vi "Eval Ping Feedback.vi"(7 "IP Address(loopback=127.0.0.1)":string="127.0.0.1", 8 "error in (no error)":errorcluster, 9 "Pings sent":i32, 10 "Ping feedback":string, 11 "object in":refnum<class "Ghetto_ping.lvclass">) -> (0 "error out":errorcluster, 1 "Report":string, 2 "Fraction returned":dbl, 3 "object out":refnum<class "Ghetto_ping.lvclass">)   [LabVIEW 2013, in "Ghetto_ping.lvclass"]
uses:
  Ghetto_ping.lvclass
panel:
  # "I AM REENTRANT"
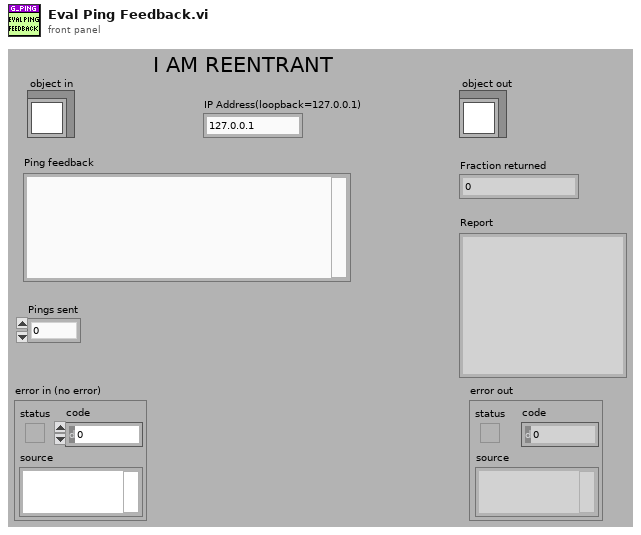
[diagram p1: front panel]
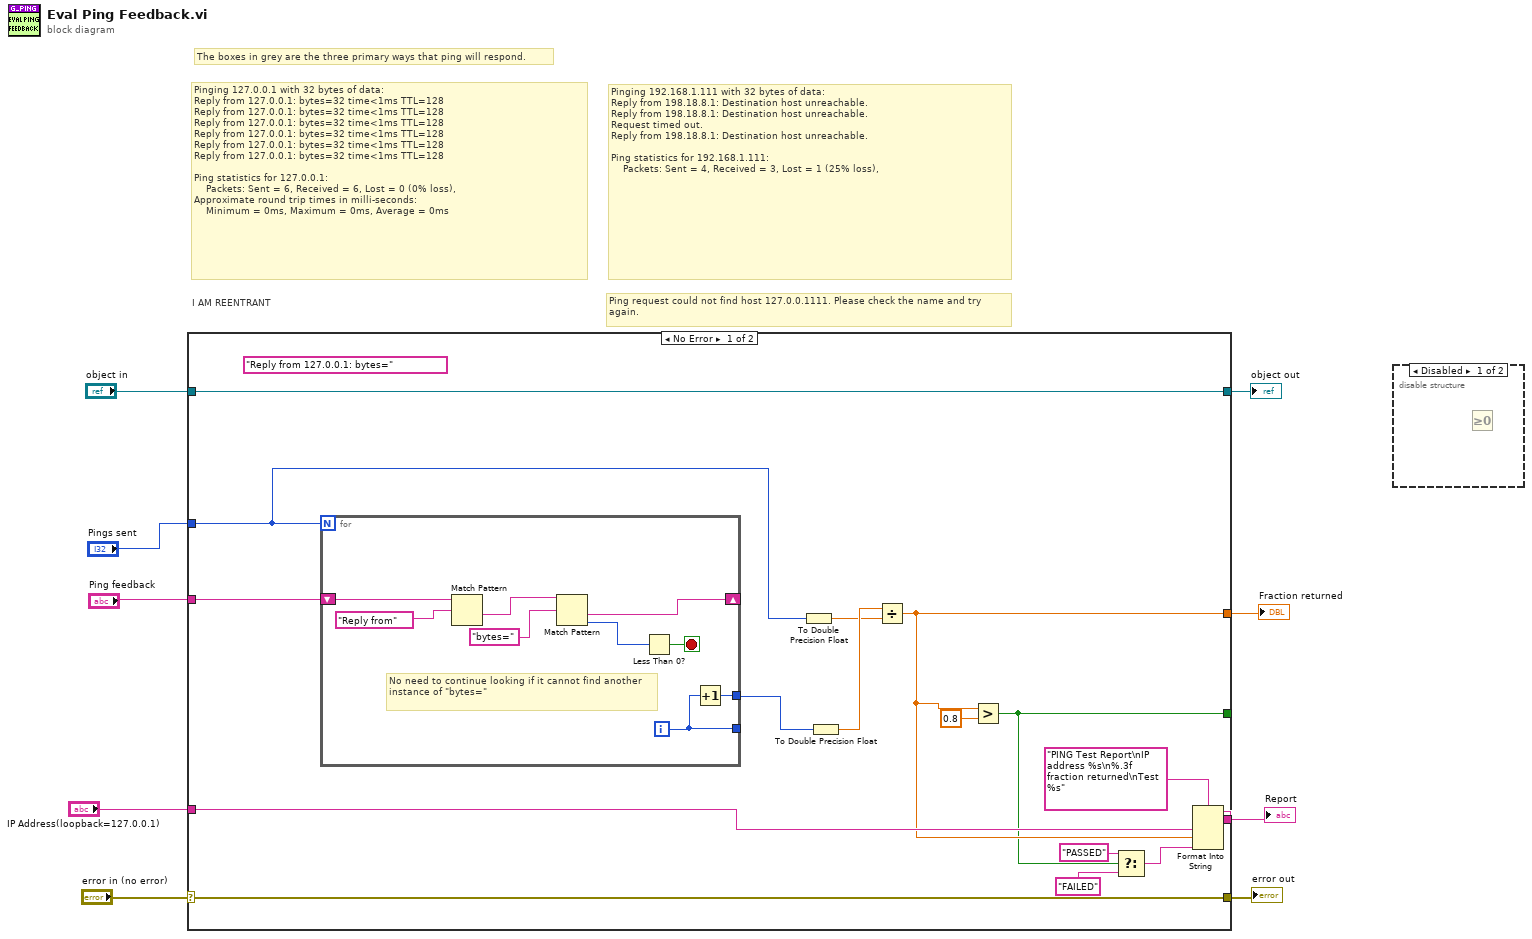
[diagram p0: block diagram]
diagram:
  # "Pinging 192.168.1.111 with 32 bytes of data:\nReply from 198.18.8.1: Destination host unreachable.\nReply from 198.18.8.1: Destination host unreachable.\nRequest timed out.\nReply from 198.18.8.1: Destination host unreachable.\n\nPing statistics for 192.168.1.111:\n    Packets: Sent = 4, Received = 3, Lost = 1 (25% loss),"
  # "The boxes in grey are the three primary ways that ping will respond."
  # "Ping request could not find host 127.0.0.1111. Please check the name and try again."
  # "Pinging 127.0.0.1 with 32 bytes of data:\nReply from 127.0.0.1: bytes=32 time<1ms TTL=128\nReply from 127.0.0.1: bytes=32 time<1ms TTL=128\nReply from 127.0.0.1: bytes=32 time<1ms TTL=128\nReply from 127.0.0.1: bytes=32 time<1ms TTL=128\nReply from 127.0.0.1: bytes=32 time<1ms TTL=128\nReply from 127.0.0.1: bytes=32 time<1ms TTL=128\n\nPing statistics for 127.0.0.1:\n    Packets: Sent = 6, Received = 6, Lost = 0 (0% loss),\nApproximate round trip times in milli-seconds:\n    Minimum = 0ms, Maximum = 0ms, Average = 0ms"
  # "I AM REENTRANT"
  n1 = case shown="No Error" "error in (no error)" {
    selector: "error in (no error)" -> [w25 w36]
    tunnel: [w25 w36] -> w8
    tunnel: [w24 w35] -> w6
    tunnel: "object in" -> [w24 w35]
    tunnel: "Pings sent" -> [w22 _]
    tunnel: "Ping feedback" -> [w23 _]
    tunnel: [w14 _] -> w3
    tunnel: [w17 _] -> w2
    tunnel: "IP Address(loopback=127.0.0.1)" -> [w16 _]
    tunnel: [w11 _] -> _
    frame No Error {
      (unwired) "Reply from 127.0.0.1: bytes="
      n2 = for {
        N: w22 -> [_]
        shift-right: [w30] -> _
        shift-left: w23 -> [w34]
        tunnel: [w27] -> _
        tunnel: [w26] -> w19
        i -> [w27]
        stop <- w29 stop-if-true
        # "No need to continue looking if it cannot find another instance of \"bytes=\""
        n3 = Match Pattern(string=w34, regular expression="Reply from") -> (after substring=w32:string)  [unwired: 1 in, 3 out]
        n4 = Match Pattern(string=w32, regular expression="bytes=") -> (after substring=w30:string, offset past match=w28:i32)  [unwired: 1 in, 2 out]
        n5 = Less Than 0?(x=w28) -> (x < 0?=w29:bool)
        n6 = Increment(x=w27) -> (x+1=w26:i32)
      }
      n7 = To Double Precision Float(number=w22) -> (double precision float=w20:dbl)
      n8 = To Double Precision Float(number=w19) -> (double precision float=w21:dbl)
      n9 = Divide(x=w21, y=w20) -> (x/y=w14:dbl)
      n10 = Greater?(x=w14, y=0.8) -> (0:w11:bool)
      n11 = Select(t="PASSED" ("format string"), s=w11, f="FAILED" ("format string")) -> (s? t:f=w10:string)
      n12 = Format Into String(format string="PING Test Report\nIP address %s\n%.3f fraction returned\nTest %s", w16, w14, w10) -> (resulting string=w17:string)  [unwired: 2 in, 1 out]
    }
    frame Error {
    }
  }
  "error out" <- w8
  "object out" <- w6
  "Fraction returned" <- w3
  "Report" <- w2
  n13 = disable-structure shown="Disabled" {
    frame Disabled {
      n14 = Greater Or Equal To 0?() -> ()  [unwired: 1 in, 1 out]
    }
    frame Enabled {
    }
  }
